vi "Entry.vi"(8 "error in (no error)":errorcluster, 11 "Idle in":refnum<class "Idle.lvclass">) -> (0 "error out":errorcluster, 3 "Idle out":refnum<class "Idle.lvclass">)   [LabVIEW 2013, in "Process States.lvlib" / "Idle.lvclass"]
doc: "This override sends a Log Event message to the UI, with the string \"Entering Idle State\" as its payload."
uses:
  Idle.lvclass
  Process State/Process State.lvclass
  <vilib>/ActorFramework/Actor/Actor.lvclass/Actor.ctl
  State Pattern UI/Log Event Msg/Log Event Msg.lvclass/Log Event Msg.ctl
  <vilib>/ActorFramework/Message Enqueuer/Message Enqueuer.lvclass/Message Enqueuer.ctl
  <vilib>/ActorFramework/Message Enqueuer/Enqueue.vi
  <vilib>/ActorFramework/Message Priority Queue/Priority Enqueue.vi
  State Pattern UI/Log Event Msg/Log Event Msg.lvclass
  <vilib>/ActorFramework/Actor/Actor.lvclass
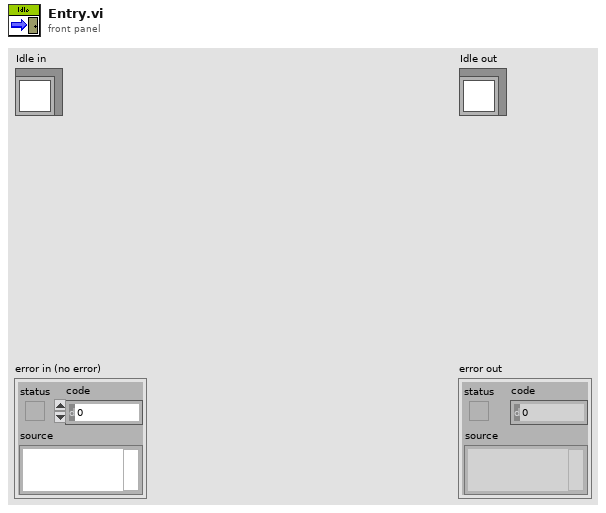
[diagram p1: front panel]
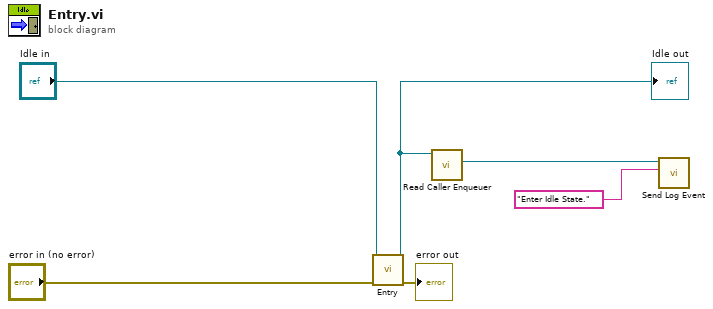
[diagram p0: block diagram]
diagram:
  n1 = call-parent "Entry.vi"("error in (no error)"="error in (no error)", "New State"="Idle in") -> ("error out"=→"error out":errorcluster, "State out"=w1:refnum<class "Idle.lvclass">)  [unwired: 8 in]
  "Idle out" <- w1
  n2 = call <vilib>:"Read Caller Enqueuer.vi"("Actor"=w1) -> ("Caller Enqueuer"=w2:refnum<class "Message Enqueuer.lvclass">)  [unwired: 10 in]
  n3 = call "Send Log Event.vi"("Event Text"="Enter Idle State.", "Message Enqueuer"=w2) -> ()  [unwired: 9 in, 1 out]
